vi "gantry_rot_query.vi"(6 "VISA resource name":refnum<visa-resource-name>) -> (0 "Motor pulse time (T/2) [us]":i32, 1 "Second char (dir is cw? 1 or 0)":string, 2 "First char (N = Not Running, R = Ramping, G = Going)":string, 3 "read buffer":string, 4 "VISA resource name out":refnum<visa-resource-name>)   [LabVIEW 2021]
panel:
  in  "microcontroller dt [us]":i32=10
  out "Third char (Motor pulse time (= speed) in units of 10us)":string
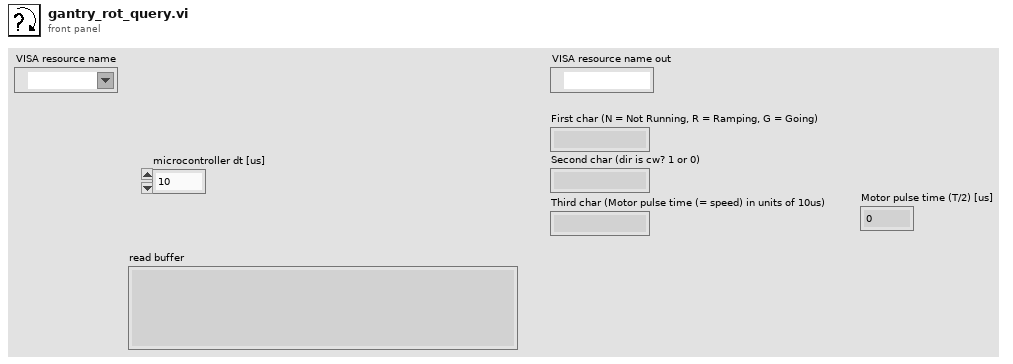
[diagram p1: front panel]
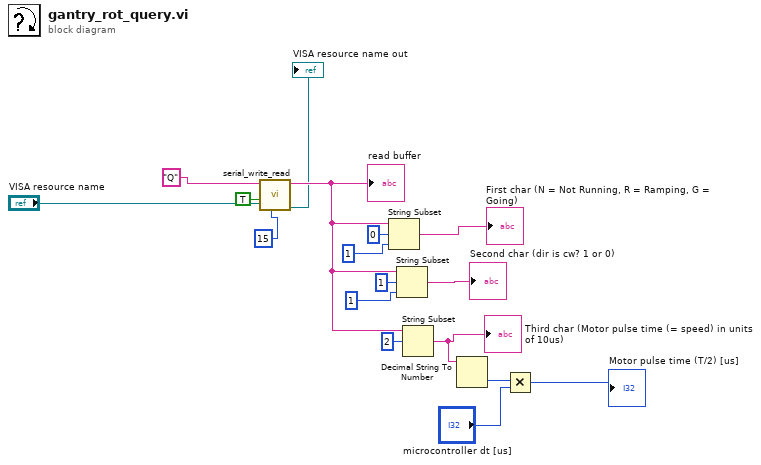
[diagram p0: block diagram]
diagram:
  n1 = call "serial_write_read.vi"("read byte count"=u32 15 ("byte count"), "VISA resource name"="VISA resource name", "Clear buffer"=TRUE, "write buffer"="Q") -> ("VISA resource name out"=→"VISA resource name out":refnum<visa-resource-name>, "read buffer"=w9:string)  [unwired: 6 in]
  "read buffer" <- w9
  n2 = String Subset(string=w9, offset (0)=0, length (rest)=1 ("length (rest)")) -> (substring=→"First char (N = Not Running, R = Ramping, G = Going)":string)
  n3 = String Subset(string=w9, offset (0)=1, length (rest)=1 ("length (rest)")) -> (substring=→"Second char (dir is cw? 1 or 0)":string)
  n4 = String Subset(string=w9, offset (0)=2) -> (substring=w7:string)  [unwired: 1 in]
  "Third char (Motor pulse time (= speed) in units of 10us)" <- w7
  n5 = Decimal String To Number(string=w7) -> (number=w6:i32)  [unwired: 2 in, 1 out]
  n6 = Multiply(x=w6, y="microcontroller dt [us]") -> (x*y=→"Motor pulse time (T/2) [us]":i32)
